vi "Get All First Level Nodes.vi"(8 "error in":errorcluster, 11 "Fast Tree in":refnum<class "Fast Tree.lvclass">) -> (0 "error out":errorcluster, 2 "Array":T1(array[cluster]), 3 "Fast Tree out":refnum<class "Fast Tree.lvclass">)   [LabVIEW 2019, in "Fast Tree.lvclass"]
uses:
  Fast Tree.lvclass
  Fast Tree.lvclass/Fast Tree.ctl
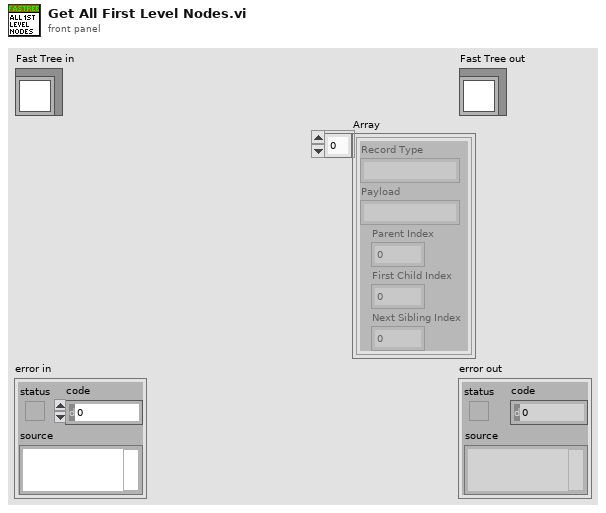
[diagram p1: front panel]
types:
  T1 = cluster{"Record Type":string, "Payload":string, "Parent Index":i32, "First Child Index":i32, "Next Sibling Index":i32}[]
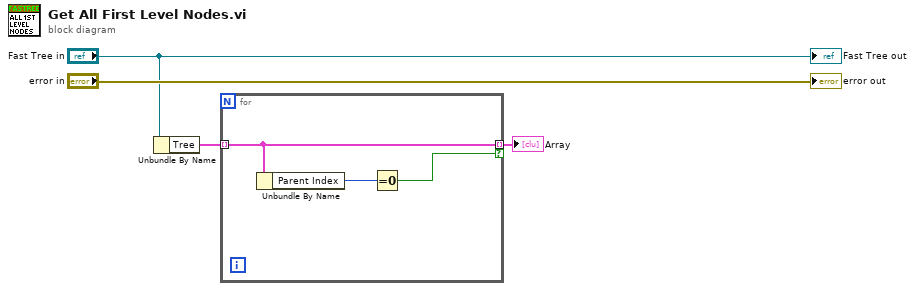
[diagram p0: block diagram]
diagram:
  n1 = Unbundle By Name("Fast Tree in") -> ("Tree"=w2:T1)
  n2 = for {
    tunnel: w2 -> [w7] mode=indexing
    tunnel: [w7] -> w1 mode=indexing if=w5
    n3 = Unbundle By Name(w7) -> ("Parent Index"=w6:i32)
    n4 = Equal To 0?(x=w6) -> (x = 0?=w5:bool)
  }
  "Array" <- w1
  "error out" <- "error in"
  "Fast Tree out" <- "Fast Tree in"
